vi "F1_Write_Config.vi"(4 "error in (no error)":errorcluster, 7 "Config Refnum":T1) -> (0 "error out":errorcluster, 3 "refnum out":T1)   [LabVIEW 2015]
uses:
  <vilib>/Utility/config.llb/Config Data RefNum.ctl
  GSP_F1_Global.vi
  <vilib>/Utility/config.llb/Write Key (I32).vi
  <vilib>/Utility/config.llb/Write Key (Double).vi
  <vilib>/Utility/config.llb/NI_LVConfig.lvlib
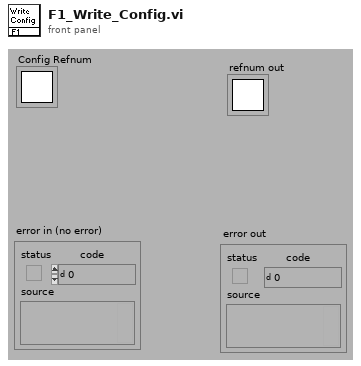
[diagram p1: front panel]
types:
  T1 = typedef "NI_LVConfig.lvlib/Config Data RefNum.ctl" = refnum<k1>
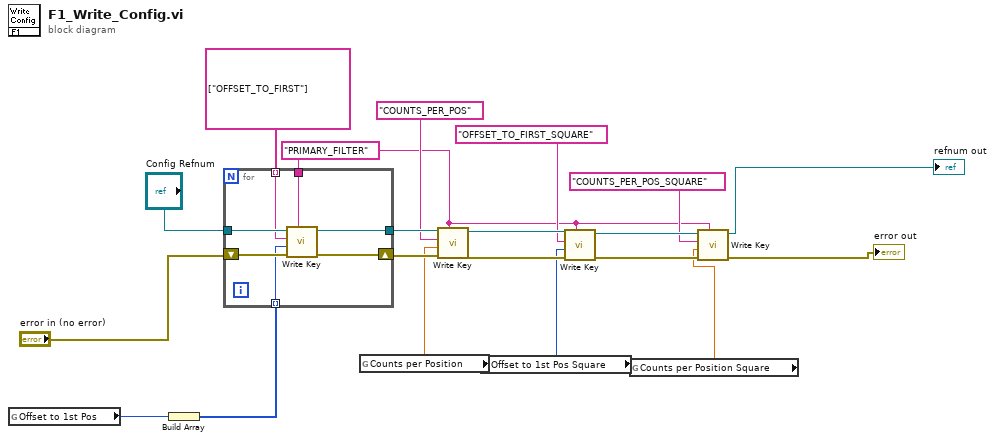
[diagram p0: block diagram]
diagram:
  w1 = "PRIMARY_FILTER"
  n1 = global read "GSP_F1_Global.vi" "Offset to 1st Pos"() -> (w14:i32)
  n2 = Build Array(w14) -> (w13:i32[])
  n3 = for {
    tunnel: "Config Refnum" -> [w26]
    shift-right: [w25] -> w16
    shift-left: "error in (no error)" -> [w27]
    tunnel: [w24] -> w17
    tunnel: string[] ["OFFSET_TO_FIRST"] -> [w23] mode=indexing
    tunnel: w1 -> [w22]
    tunnel: w13 -> [w21] mode=indexing
    n4 = call-poly <vilib>:"Write Key.vi"("section"=w22, "error in (no error)"=w27, "value"=w21, "key"=w23, "refnum"=w26) -> ("error out"=w25:errorcluster, "refnum out"=w24:T1)  [unwired: 4 in, 1 out]
  }
  n5 = global read "GSP_F1_Global.vi" "Counts per Position"() -> (w12:dbl)
  n6 = call-poly <vilib>:"Write Key.vi"("section"=w1, "error in (no error)"=w16, "value"=w12, "key"="COUNTS_PER_POS", "refnum"=w17) -> ("error out"=w6:errorcluster, "refnum out"=w11:T1)  [unwired: 4 in, 1 out]
  n7 = global read "GSP_F1_Global.vi" "Offset to 1st Pos Square"() -> (w5:i32)
  n8 = call-poly <vilib>:"Write Key.vi"("section"=w1, "error in (no error)"=w6, "value"=w5, "key"="OFFSET_TO_FIRST_SQUARE", "refnum"=w11) -> ("error out"=w7:errorcluster, "refnum out"=w10:T1)  [unwired: 4 in, 1 out]
  n9 = global read "GSP_F1_Global.vi" "Counts per Position Square"() -> (w4:dbl)
  n10 = call-poly <vilib>:"Write Key.vi"("section"=w1, "error in (no error)"=w7, "value"=w4, "key"="COUNTS_PER_POS_SQUARE", "refnum"=w10) -> ("error out"=→"error out":errorcluster, "refnum out"=→"refnum out":T1)  [unwired: 4 in, 1 out]
